vi "DIO.vi"(0 "System no.":i32=1 min=1 max=4 step=1, 2 "DO's to command":string[](array[string]), 3 "DO mode":bool[](array[boolean]), 5 "error in":errorcluster, 6 "DO mode format":enum16{"boolean", "hexadecimal", "decimal"}(ring), 7 "DO pattern":u32 format="%x") -> (19 "error out":errorcluster)   [LabVIEW 2020]
doc: "Switches digital outputs on or off. For DO mode format = Boolean, DO mode must be selected for each DO to command. For DO mode format = hexadecimal (decimal), DO mode and DO's to command are not valid and DO pattern must be selected correctly in hexadecimal (decimal) format. \n\nC-413: DO mode format is Boolean, DO's to command can be 1 to 5. DO pattern is not valid.\n\nC-702, C-843, C-843.PM, C-848: DO's to command can be A-H. DO mode format is Boolean, DO pattern is not valid.\n\nC-865, C-866: DO's to command can be A-B. . DO mode format is Boolean, DO pattern is not valid.\n\nC-867, C-891, E-861, E-871, E-873, E-874, Mercury_GCS: For DO mode format = Boolean, DO's to command can be 1-4 and only one DO per command allowed. For DO mode format = hexadecimal, DO's to command and DO mode are not valid and DO pattern must be set correctly (all DO's are set with one single command).\n\nC-877: For DO mode format = Boolean, DO's to command can be 1-4 and only one DO per command allowed. For DO mode format = hexadecimal, DO's to command and DO mode are not valid and DO pattern must be set correctly (all DO's are set with one single command).Check HLP? answer to find out if DIO is supported\n\nC-884: For DO mode format = Boolean, DO's to command can be 1 to 4. Up to four DO's per command call are allowed. For DO mode format = hexadecimal, DO's to command and DO mode are not valid and DO pattern must be set correctly (all DO's are set with one single command). \n\nC-880: DO's to command can be A-H (one C-842 inside), A-P (two C-842 inside) etc. DO mode format is Boolean, DO pattern is not valid.\n\nF-206, M-8X0: For DO mode format = Boolean, DO's to command can be 1 to 8. For DO mode format = hexadecimal, DO's to command and DO mode are not valid and DO pattern must be set correctly (all DO's are set with one single command). Only for GCS syntax version = GCS 2.0 or higher (Check with CSV?.vi. If CSV?.vi is not supported, syntax version is GCS 1.0).\n\nHydra: For DO mode format = Boolean, DO's to command can be 1-3 and only one DO per command allowed. For DO mode format = hexadecimal, DO's to command and DO mode are not valid and DO pattern must be set correctly (all DO's are set with one single command). \n\nMercury: DO's to command can be A-D, E-H, I-L etc., see GCS DLL Manual for details. DO mode format is Boolean, DO pattern is not valid."
panel:
  # "Switches digital outputs on or off."
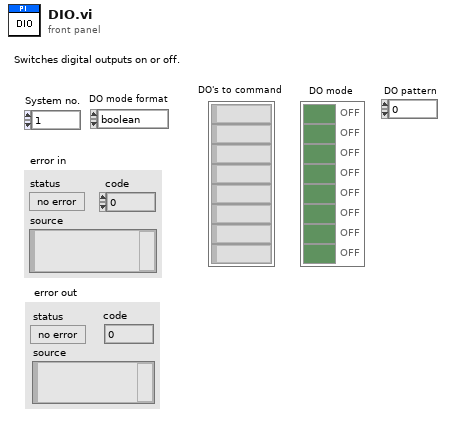
[diagram p1: front panel]
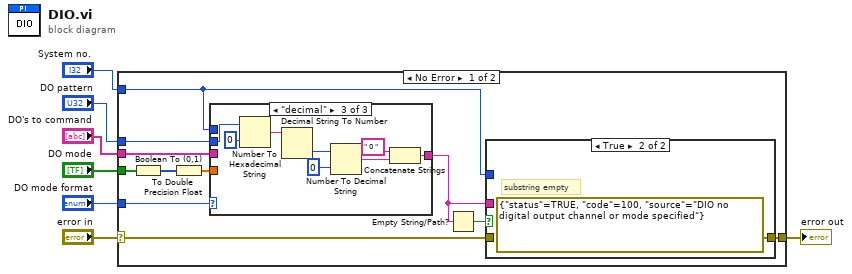
[diagram p0: block diagram]
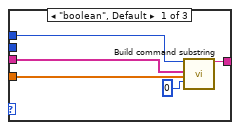
[diagram p2: hidden frame]
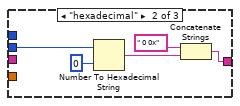
[diagram p3: hidden frame]
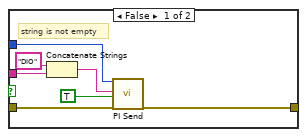
[diagram p4: hidden frame]
diagram:
  n1 = case shown="No Error" "error in" {
    selector: "error in" -> [w8 w45]
    tunnel: [w18 w45] -> w7
    tunnel: "DO's to command" -> [w17 _]
    tunnel: "DO mode" -> [w16 _]
    tunnel: "System no." -> [w13 _]
    tunnel: "DO mode format" -> [w12 _]
    tunnel: "DO pattern" -> [w11 _]
    frame No Error {
      n2 = Boolean To (0,1)(Boolean=w16) -> (0, 1=w15:i16[])
      n3 = To Double Precision Float(number=w15) -> (double precision float=w14:dbl[])
      n4 = case shown="\"decimal\"" w12 {
        tunnel: [w23 w24 w35] -> w9
        tunnel: w17 -> [w22 _ _]
        tunnel: w14 -> [w20 _ _]
        tunnel: w13 -> [w19 _ _]
        tunnel: w11 -> [_ w28 w31]
        frame "boolean", Default {
          n5 = call "Build command substring.vi"("System no."=w19, "Affected axes"=w22, "Parameters"=w20, "No. of digits"=i16 0 ("No.of digits")) -> ("Command substring"=w23:string)  [unwired: 3 in, 12 out]
        }
        frame "hexadecimal" {
          n6 = Number To Hexadecimal String(1:i16 0 ("width (-)"), 2:w28) -> (0:w25:string)
          n7 = Concatenate Strings(" 0 0x" ("string"), w25) -> (w24:string)
        }
        frame "decimal" {
          n8 = Number To Hexadecimal String(1:i16 0 ("width (-)"), 2:w31) -> (0:w33:string)
          n9 = Decimal String To Number(string=w33) -> (number=w34:i32)  [unwired: 3 out]
          n10 = Number To Decimal String(number=w34, width (-)=i16 0) -> (decimal integer string=w32:string)
          n11 = Concatenate Strings(" 0 " ("string"), w32) -> (w35:string)
        }
      }
      n12 = Empty String/Path?(string/path=w9) -> (empty?=w10:bool)
      n13 = case shown="True" w10 {
        tunnel: w9 -> [w42 _]
        tunnel: [w38 errorcluster {"status"=TRUE, "code"=100, "source"="DIO no digital output channel or mode specified"} ("error out")] -> w18
        tunnel: w8 -> [w39 _]
        tunnel: w13 -> [w37 _]
        frame False {
          # "string is not empty"
          n14 = Concatenate Strings("DIO", w42) -> (w40:string)
          n15 = call "PI Send.vi"("System no."=w37, "String to send"=w40, "Attach termination char.?"=TRUE ("Attach Linefeed?"), "error in"=w39) -> ("error out"=w38:errorcluster)  [unwired: 2 in, 13 out]
        }
        frame True {
          # "substring empty"
        }
      }
    }
    frame Error {
    }
  }
  "error out" <- w7
